vi "Check Status.vi"(0 "session in":T4[](array[typedef]) {"rx baseband session"."3630 session"."Address Space" items=["VXI/VME A16"=1, "VXI/VME A24"=2, "VXI/VME A32"=3, "VXI/VME A64"=4, "PXI Memory Allocations"=9, "PXI Configuration"=10, "PXI BAR0"=11, "PXI BAR1"=12, "PXI BAR2"=13, "PXI BAR3"=14, "PXI BAR4"=15, "PXI BAR5"=16]; "tx baseband session"."3610 session"."Address Space" items=["VXI/VME A16"=1, "VXI/VME A24"=2, "VXI/VME A32"=3, "VXI/VME A64"=4, "PXI Memory Allocations"=9, "PXI Configuration"=10, "PXI BAR0"=11, "PXI BAR1"=12, "PXI BAR2"=13, "PXI BAR3"=14, "PXI BAR4"=15, "PXI BAR5"=16]}, 11 "error in":errorcluster) -> (4 "session out":T4[](array[typedef]) {"rx baseband session"."3630 session"."Address Space" items=["VXI/VME A16"=1, "VXI/VME A24"=2, "VXI/VME A32"=3, "VXI/VME A64"=4, "PXI Memory Allocations"=9, "PXI Configuration"=10, "PXI BAR0"=11, "PXI BAR1"=12, "PXI BAR2"=13, "PXI BAR3"=14, "PXI BAR4"=15, "PXI BAR5"=16]; "tx baseband session"."3610 session"."Address Space" items=["VXI/VME A16"=1, "VXI/VME A24"=2, "VXI/VME A32"=3, "VXI/VME A64"=4, "PXI Memory Allocations"=9, "PXI Configuration"=10, "PXI BAR0"=11, "PXI BAR1"=12, "PXI BAR2"=13, "PXI BAR3"=14, "PXI BAR4"=15, "PXI BAR5"=16]}, 6 "rx status":T3(array[cluster]), 8 "tx status":T1(array[cluster]), 10 "dac alarms":T2[][](array[typedef]), 15 "error out":errorcluster)   [LabVIEW 2019, in "mmWave HW Control.lvlib"]
uses:
  Low-level/TypeDefs/Session.ctl
  <instrlib>/niMmWave/ni3620/Config/v1/Host/Public/High-Level/niMmWave Session.ctl
  <instrlib>/_niInstr/Register Bus/v0/Host/Public/Register Bus Session.ctl
  <instrlib>/_niInstr/Register Bus/v0/Host/Private/Session Data.ctl
  <instrlib>/niMmWave/ni3620/Config/v1/Host/Public/Typedefs/Board Information.ctl
  <instrlib>/niMmWave/ni3620/Config/v1/Host/Public/Typedefs/Hardware Revision.ctl
  <instrlib>/niMmWave/ni3620/Config/v1/Host/Public/Typedefs/Gain Mapping.ctl
  <instrlib>/niMmWave/ni3620/Config/v1/Host/Public/Typedefs/Correction Data.ctl
  <instrlib>/niMmWave/ni3620/Config/v1/Host/Public/Typedefs/Opera Characterization.ctl
  <instrlib>/niMmWave/ni3620/Config/v1/Host/Public/Corrections/Typedefs/Opera Characterization Main Header.ctl
  <instrlib>/niMmWave/ni3620/Config/v1/Host/Public/Corrections/Typedefs/Opera IF Board Information.ctl
  <instrlib>/niMmWave/ni3620/Config/v1/Host/Public/Corrections/Typedefs/Opera Characterization Instance Header.ctl
  <instrlib>/niMmWave/ni3620/Config/v1/Host/Public/Corrections/Typedefs/Opera Characterization Device Data Header.ctl
  <instrlib>/niMmWave/ni3620/Config/v1/Host/Public/Corrections/Typedefs/Opera LO Characterization Data Header.ctl
  <instrlib>/niMmWave/ni3620/Config/v1/Host/Public/Corrections/Typedefs/Opera IF Board Characterization Data Header.ctl
  <instrlib>/niMmWave/ni3620/Config/v1/Host/Public/Corrections/Typedefs/Opera Characterization Device Data.ctl
  <instrlib>/niMmWave/ni3620/Config/v1/Host/Public/Corrections/Typedefs/Opera LO2 Board Characterization Data.ctl
  <instrlib>/niMmWave/ni3620/Config/v1/Host/Public/Corrections/Typedefs/Opera LO Characterization Data.ctl
  <instrlib>/niMmWave/ni3620/Config/v1/Host/Public/Corrections/Typedefs/Opera IF Board Characterization Data.ctl
  <instrlib>/niMmWave/ni3620/Config/v1/Host/Public/Corrections/Typedefs/Opera IQ Impairment Data.ctl
  <instrlib>/niMmWave/ni3620/Config/v1/Host/Public/Typedefs/mmWave Adapter Session Data.ctl
  <instrlib>/niMmWave/ni3620/Config/v1/Host/Public/Typedefs/mmWave Adapter Data.ctl
  <instrlib>/niMmWave/ni3620/Config/v1/Host/Public/Typedefs/mmWave Adapter 2.ctl
  <instrlib>/niMmWave/ni3620/Config/v1/Shared/Typedefs/Subsystem ID.ctl
  <instrlib>/niMmWave/ni3620/Config/v1/Host/Public/Typedefs/mmWave Adapter Channel Information.ctl
  <instrlib>/niMmWave/ni3620/Config/v1/Host/Public/Typedefs/Temperature Coefficients.ctl
  <instrlib>/niMmWave/ni3620/Config/v1/Host/Public/Typedefs/mmWave Characterization.ctl
  <instrlib>/niMmWave/ni3620/Config/v1/Host/Public/Corrections/Typedefs/mmWave Characterization Main Header.ctl
  <instrlib>/niMmWave/ni3620/Config/v1/Host/Public/Corrections/Typedefs/mmWave Characterization Instance Header.ctl
  <instrlib>/niMmWave/ni3620/Config/v1/Host/Public/Typedefs/Session Cache.ctl
  <instrlib>/niMmWave/ni3620/Config/v1/Host/Public/Typedefs/LO2 settings cache.ctl
  <instrlib>/niMmWave/ni3620/Config/v1/Host/Public/Typedefs/LO2 source.ctl
  <instrlib>/niMmWave/ni3620/Config/v1/Host/Public/Typedefs/Desired and Coerced.ctl
  <instrlib>/niMmWave/ni3620/Config/v1/Host/Public/Typedefs/Export cache.ctl
  <instrlib>/niMmWave/ni3620/Config/v1/Host/Public/Typedefs/Path cache.ctl
  <instrlib>/niMmWave/ni3620/Config/v1/Host/Public/Typedefs/Daughterboard Type.ctl
  <instrlib>/niMmWave/ni3620/Config/v1/Host/Public/Typedefs/LO1 settings cache.ctl
  <instrlib>/niMmWave/ni3620/Config/v1/Host/Public/Typedefs/LO1 Source.ctl
  <instrlib>/niMmWave/ni3620/Config/v1/Host/Public/Typedefs/mmWave export cache.ctl
  <instrlib>/niMmWave/ni3620/Config/v1/Host/Private/Board/LO2/LO2 Board Configuration Cache.ctl
  <instrlib>/niMmWave/ni3620/Config/v1/Host/Public/Typedefs/reference clock routing settings.ctl
  <instrlib>/niMmWave/ni3620/Config/v1/Host/Public/Typedefs/LO2 routing settings.ctl
  <instrlib>/niMmWave/ni3620/Config/v1/Host/Private/Board/LO1/LO1 Board Configuration Cache.ctl
  <instrlib>/niMmWave/ni3620/Config/v1/Host/Public/Typedefs/LO1 source settings.ctl
  <instrlib>/niMmWave/ni3620/Config/v1/Host/Public/Typedefs/LO1 export settings.ctl
  <instrlib>/niMmWave/ni3620/Config/v1/Host/Public/Typedefs/LO1 mmWave settings.ctl
  Low-level/TypeDefs/Tx Baseband Session.ctl
  <instrlib>/niMmWave/ni3610 and ni3630/controls/public/Main Settings.ctl
  <vilib>/Instr/_visa.llb/VISA Register Access Address Space.ctl
  <instrlib>/niMmWave/ni3610 and ni3630/controls/public/Register Adresses.ctl
  <instrlib>/niMmWave/ni3610 and ni3630/controls/public/Base Card Type.ctl
  <instrlib>/niMmWave/ni3610 and ni3630/controls/private/IQ Card Revision.ctl
  <instrlib>/niMmWave/ni3610 and ni3630/controls/public/Board Capability.ctl
  Low-level/TypeDefs/Blank FPGA Reference.ctl
  Low-level/TypeDefs/Rx Baseband Session.ctl
  Low-level/TypeDefs/Hardware Configuration.ctl
  Low-level/TypeDefs/Direction.ctl
  Low-level/TypeDefs/Gain Ranging.ctl
  Low-level/TypeDefs/PXI Trigger Bus Info.ctl
  <instrlib>/niMmWave/ni3610 and ni3630/controls/public/DAC Alarms.ctl
  Low-level/TypeDefs/RX FPGA Reference.ctl
  <instrlib>/niMmWave/ni3610 and ni3630/controls/public/Converter Path Selector.ctl
  Low-level/TypeDefs/TX FPGA Reference.ctl
  <vilib>/rvi/errors/niLvFpgaAdjustHostInterfaceError.vi
  <vilib>/rvi/interface/nirviReadWriteControl/nirviReadWriteControl.xnode
  mmWave HW Control.lvlib
  NiFpgaLv.dll
  <vilib>/rvi/interface/Simulation/niFpgaSimulationCallBeginRW.vi
  <instrlib>/niMmWave/ni3610 and ni3630/ni3610_and_ni3630_Driver_Lib.lvlib
  <instrlib>/niMmWave/ni3620/Config/v1/Host/niMmWave Config v1 Host.lvlib
  <instrlib>/_niInstr/Register Bus/v0/Host/niInstr Register Bus v0 Host.lvlib
  <instrlib>/niMmWave/ni3620/Config/v1/Shared/niMmWave Config v1 Shared.lvlib
panel:
  # "Lane Number"
  # "0     1     2    3     4    5     6    7"
  # "Multiframe Alignment Error"
  # "Frame Alignment Error"
  # "Link Configuration Error"
  # "Elastic Buffer Overflow"
  # "Elastic Buffer Match Error"
  # "Code Group Synch. Error"
  # "8b/10b Not-in-Table Error"
  # "8b/10b Disparity Error"
  # "Lane Number"
  # "0     1     2    3     4    5     6    7"
  # "FIFO Write Error"
  # "FIFO Write Full"
  # "FIFO Read Error"
  # "FIFO Read Empty"
  # "Short Test Error"
  # "LOS Detect Alarm"
  # "SYSREF Alarms\n0      1      2     3"
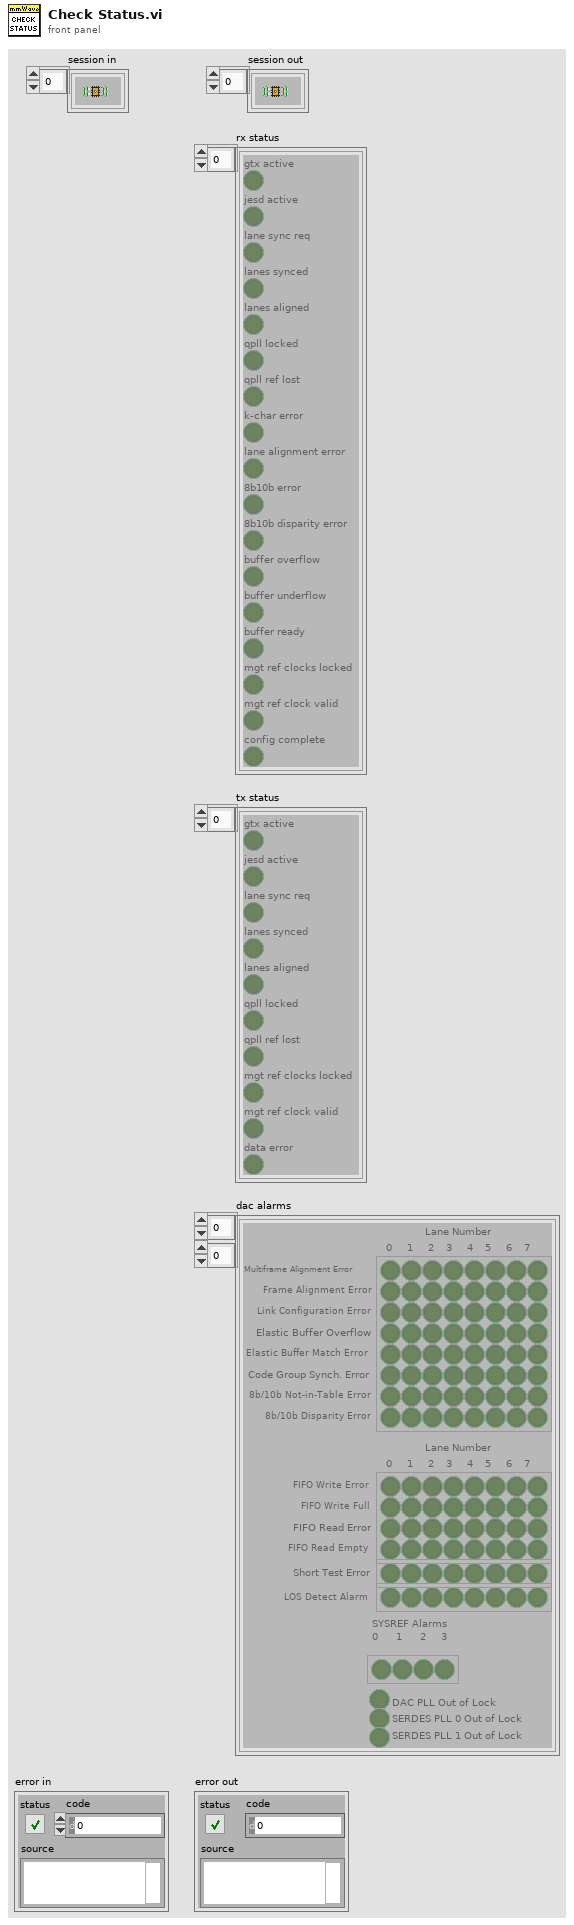
[diagram p1: front panel]
types:
  T1 = cluster{"gtx active":bool, "jesd active":bool, "lane sync req":bool, "lanes synced":bool, "lanes aligned":bool, "qpll locked":bool, "qpll ref lost":bool, "mgt ref clocks locked":bool, "mgt ref clock valid":bool, "data error":bool}[]
  T2 = typedef "ni3610_and_ni3630_Driver_Lib.lvlib/DAC Alarms.ctl" = cluster{"Lane Errors":bool[][], "FIFO Errors":bool[][], "Short Test Alarms":bool[], "LOS Alarms":bool[], "SYSREF Errors":bool[], "DAC38J84 PLL Out of Lock 3":bool, "DAC38J84 RW0 Out of Lock 3":bool, "DAC38J84 RW1 Out of Lock 3":bool}
  T3 = cluster{"gtx active":bool, "jesd active":bool, "lane sync req":bool, "lanes synced":bool, "lanes aligned":bool, "qpll locked":bool, "qpll ref lost":bool, "k-char error":bool, "lane alignment error":bool, "8b10b error":bool, "8b10b disparity error":bool, "buffer overflow":bool, "buffer underflow":bool, "buffer ready":bool, "mgt ref clocks locked":bool, "mgt ref clock valid":bool, "config complete":bool}[]
  T4 = typedef "Session.ctl" = cluster{"3620 session":refnum<queue>, "tx baseband session":T5, "rx baseband session":T13, "tx gain (dB)":dbl, "rx gain (dB)":dbl, "hardware configuration":T14, "gain ranging":T16[], "pxi trigger bus information":T17}
  T5 = typedef "Tx Baseband Session.ctl" = cluster{"3610 session":T6, "7902 reference":T12}
  T6 = typedef "ni3610_and_ni3630_Driver_Lib.lvlib/Main Settings.ctl" = cluster{"VISA resource name":refnum<visa-resource-name>, "Address Space":T7, "window_offset":u32, "register_addresses":T8, "required_MM_fpga_version":cluster{"signature":u32, "hardware":u32, "current revision":u32, "oldest revision":u32}, "CPLD Oldest Compat Version ":cluster{"hardware":u32, "CPLD firmware":u32}, "MM_FPGA_image_location":string, "is_init":bool, "card_type":T9, "DacLmkConfigFileName":string, "AdcLmkConfigFileName":string, "AdcConfigFileName":string, "DacConfigFileName_RevA":string, "DacConfigFileName_RevB":string, "Mulde hardware revision":u8, "bypass DAC PLL\n":bool, "IQ Card Revision":T10, "board capability":T11}
  T7 = typedef "VISA Register Access Address Space.ctl" = u16
  T8 = typedef "ni3610_and_ni3630_Driver_Lib.lvlib/Register Adresses.ctl" = cluster{"MM based Registers":cluster{"Revision":u32, "OldestCompatRev":u32, "signature":u32, "scratch":u32, "LedControl":u32, "BoardHwRev":u32, "BoardControl":u32, "ThermalStatus":u32, "BasebandStatus":u32, "BasebandControl":u32, "BasebandAuxSetup":u32, "BasebandAuxStatus":u32, "LmkSyncOutSetup":u32, " AdcSyncOutSetup":u32, " InjSyncOutSetup":u32, " PxiTrig0OutSetup":u32, " PxiTrig1OutSetup":u32, " PxiTrig2OutSetup":u32, " PxiTrig3OutSetup":u32, " PxiTrig4OutSetup":u32, " PxiTrig5OutSetup":u32, " PxiTrig6OutSetup":u32, " PxiTrig7OutSetup":u32}, "CPLD based Registers":cluster{"SlaveSignature":u32, "SlaveRevision":u32, "SlaveOldestCompatRev":u32, "SlaveScratch":u32, "SlaveSetup":u32, "SlaveStatus":u32, "IDacReg_offset":u32, "LMKRegGrp0_offset":u32, "QDacReg_offset":u32, "BrdTempSensorVal":u32, "TempSensorPowerDown":u32, "GPIOReg_offset":u32, "IAdcReg_offset":u32, "QAdcReg_offset":u32, "LMKRegGrp1_offset":u32, "QadcTempSensorVal":u32, "IadcTempSensorVal":u32, "RevisionReg":u32, "VcxoReg":u32, "CpldStatusReg":u32, "PowerReg":u32, "VBiasEnReg":u32, "ExtRefOeReg":u32, "QdacCtrlReg":u32, "QdacStatusReg":u32, "IdacCtrlReg":u32, "IdacStatusReg":u32, "QdacJtagIn":u32, "QdacJtagOut":u32, "IdacJtagIn":u32, "IdacJtagOut":u32, "IqDcSetupReg":u32, "QadcStatusReg":u32, "IadcStatusReg":u32, "BrdSetupReg":u32, "IqDcRevisionReg":u32, "PllStatusReg":u32, "EndpointScratchReg":u32, "AdcSyncCfgReg":u32, "IqCardOpampReg":u32}, "CPLD Register Offset":u32, "MM  Register Offset":u32, " PxiTrig0OutSetup":u32}
  T9 = typedef "ni3610_and_ni3630_Driver_Lib.lvlib/Base Card Type.ctl" = enum16{"unspecified", "ADC", "DAC"}
  T10 = typedef "ni3610_and_ni3630_Driver_Lib.lvlib/IQ Card Revision.ctl" = enum16{"RevA", "RevB", "RevC", "RevD"}
  T11 = typedef "ni3610_and_ni3630_Driver_Lib.lvlib/Board Capability.ctl" = cluster{"baseband sync":enum16{"no baseband sync", "baseband sync"}}
  T12 = typedef "Blank FPGA Reference.ctl" = refnum<k20>
  T13 = typedef "Rx Baseband Session.ctl" = cluster{"3630 session":T6, "7902 reference":T12}
  T14 = typedef "Hardware Configuration.ctl" = cluster{"direction":T15, "baseband only":bool}
  T15 = typedef "Direction.ctl" = enum16{"Transceiver", "Receiver", "Transmitter"}
  T16 = typedef "Gain Ranging.ctl" = cluster{"gain ranging active scope":string, "gain ranging stream session":refnum<k20>}
  T17 = typedef "PXI Trigger Bus Info.ctl" = cluster{"chassis resource name":refnum<visa-resource-name>, "7902R (TX)":i16, "3610 (TX)":i16, "3620 (IF)":i16, "3630 (RX)":i16, "7902R (RX)":i16}
  T18 = cluster{"gtx active":bool, "jesd active":bool, "lane sync req":bool, "lanes synced":bool, "lanes aligned":bool, "qpll locked":bool, "qpll ref lost":bool, "k-char error":bool, "lane alignment error":bool, "8b10b error":bool, "8b10b disparity error":bool, "buffer overflow":bool, "buffer underflow":bool, "buffer ready":bool, "mgt ref clocks locked":bool, "mgt ref clock valid":bool, "config complete":bool}
  T19 = typedef "RX FPGA Reference.ctl" = refnum<k20>
  T20 = cluster{"gtx active":bool, "jesd active":bool, "lane sync req":bool, "lanes synced":bool, "lanes aligned":bool, "qpll locked":bool, "qpll ref lost":bool, "mgt ref clocks locked":bool, "mgt ref clock valid":bool, "data error":bool}
  T21 = typedef "TX FPGA Reference.ctl" = refnum<k20>
  T22 = typedef "ni3610_and_ni3630_Driver_Lib.lvlib/Converter Path Selector.ctl" = enum16{"I-path device", "Q-path device"}
  T23 = typedef "ni3610_and_ni3630_Driver_Lib.lvlib/ADC Status.ctl" = cluster{"JESD Link Up":bool, "JESD Sync Status":bool, "JESD Realigned":bool, "JESD Aligned":bool, "Powered Down":bool, "Gain_FS[mVp-p]":dbl, "Offset_FS[mV]":dbl}
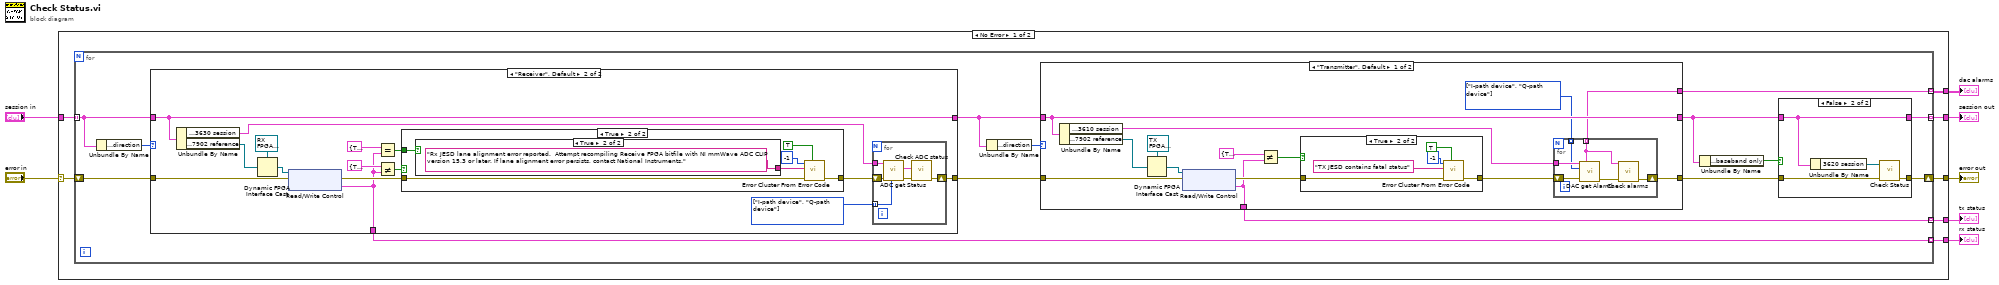
[diagram p0: block diagram]
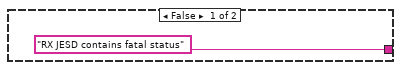
[diagram p4: hidden frame]
diagram:
  n1 = case shown="No Error" "error in" {
    selector: "error in" -> [w12 w95]
    tunnel: "session in" -> [w14 w96]
    tunnel: [w13 w96] -> w6
    tunnel: [w11 w95] -> w4
    tunnel: [w10 _] -> w3
    tunnel: [w9 _] -> w1
    tunnel: [w8 _] -> w2
    frame No Error {
      n2 = for {
        tunnel: w14 -> [w26] mode=indexing
        tunnel: [w15] -> w13 mode=indexing
        shift-right: [w19] -> w11
        shift-left: w12 -> [w28]
        tunnel: [w27] -> w10 mode=indexing
        tunnel: [w21] -> w9 mode=indexing
        tunnel: [w20] -> w8 mode=indexing
        n3 = Unbundle By Name(w26) -> ("hardware configuration.direction"=w25:T15)
        n4 = case shown="\"Receiver\", Default" w25 {
          tunnel: w26 -> [w30 w41]
          tunnel: w28 -> [w29 w45]
          tunnel: [w29 w37] -> w24
          tunnel: [_ w32] -> w27
          tunnel: [w30 w41] -> w22
          frame "Transmitter" {
          }
          frame "Receiver", Default {
            w35 = T22[] [enum."I-path device", enum."Q-path device"] items=["I-path device", "Q-path device"]
            n5 = Unbundle By Name(w41) -> ("rx baseband session.3630 session"=w36:T6, "rx baseband session.7902 reference"=w44:T12)
            n6 = Dynamic FPGA Interface Cast(Session In=T19 refnum ("fpga reference"), Type=w44) -> (Session Out=w42:T19)
            n7 = xnode "Read/Write Control"("FPGA VI Reference In"=w42, "error in"=w45) -> ("error out"=w40:errorcluster, "rxjesd.status"=w32:T18)  [unwired: 1 out]
            n8 = Equal?(x=T18 {"gtx active"=TRUE, "jesd active"=TRUE, "lane sync req"=FALSE, "lanes synced"=TRUE, "lanes aligned"=TRUE, "qpll locked"=TRUE, "qpll ref lost"=FALSE, "k-char error"=FALSE, "lane alignment error"=TRUE, "8b10b error"=FALSE, "8b10b disparity error"=FALSE, "buffer overflow"=FALSE, "buffer underflow"=FALSE, "buffer ready"=TRUE, "mgt ref clocks locked"=TRUE, "mgt ref clock valid"=TRUE, "config complete"=TRUE} ("rxjesd.status"), y=w32) -> (x = y?=w31:bool)
            n9 = Not Equal?(x=T18 {"gtx active"=TRUE, "jesd active"=TRUE, "lane sync req"=FALSE, "lanes synced"=TRUE, "lanes aligned"=TRUE, "qpll locked"=TRUE, "qpll ref lost"=FALSE, "k-char error"=FALSE, "lane alignment error"=FALSE, "8b10b error"=FALSE, "8b10b disparity error"=FALSE, "buffer overflow"=FALSE, "buffer underflow"=FALSE, "buffer ready"=TRUE, "mgt ref clocks locked"=TRUE, "mgt ref clock valid"=TRUE, "config complete"=TRUE} ("rxjesd.status"), y=w32) -> (x != y?=w39:bool)
            n10 = case shown="True" w39 {
              tunnel: w40 -> [w46 w52]
              tunnel: [w46 w51] -> w38
              tunnel: w31 -> [_ w47]
              frame False {
              }
              frame True {
                n11 = case shown="True" w47 {
                  tunnel: ["RX JESD contains fatal status" ("error message (\"\")") "Rx JESD lane alignment error reported.  Attempt recompiling Receive FPGA bitfile with NI mmWave ADC CLIP version 15.3 or later. If lane alignment error persists, contact National Instruments." ("error message (\"\")")] -> w48
                  frame False {
                  }
                  frame True {
                  }
                }
                n12 = call <vilib>:"Error Cluster From Error Code.vi"("show call chain? (False)"=TRUE, "error in (no error)"=w52, "error message (\"\")"=w48, "error code (0)"=-1 ("specific error code to clear (0: all)")) -> ("error out"=w51:errorcluster)  [unwired: 5 in]
              }
            }
            n13 = for {
              tunnel: w36 -> [w56]
              shift-right: [w58] -> w37
              shift-left: w38 -> [w60]
              tunnel: w35 -> [w55] mode=indexing
              n14 = call <instrlib>:"ADC get Status.vi"("Converter Selection"=w55, "error in"=w60, "Board Settings in"=w56) -> ("error out"=w59:errorcluster, "ADC Status"=w57:T23)  [unwired: 6 in, 1 out]
              n15 = call "Check ADC status.vi"("ADC Status"=w57, "error in (no error)"=w59) -> ("error out"=w58:errorcluster)  [unwired: 13 in]
            }
          }
        }
        n16 = Unbundle By Name(w22) -> ("hardware configuration.direction"=w23:T15)
        n17 = case shown="\"Transmitter\", Default" w23 {
          tunnel: w24 -> [w77 w93]
          tunnel: w22 -> [w76 w94]
          tunnel: [w71 _] -> w21
          tunnel: [w76 w94] -> w16
          tunnel: [w75 w93] -> w18
          tunnel: [w73 _] -> w20
          frame "Transmitter", Default {
            w74 = T22[] [enum."I-path device", enum."Q-path device"] items=["I-path device", "Q-path device"]
            n18 = Unbundle By Name(w76) -> ("tx baseband session.3610 session"=w68:T6, "tx baseband session.7902 reference"=w79:T12)
            n19 = Dynamic FPGA Interface Cast(Session In=T21 refnum ("Refnum in"), Type=w79) -> (Session Out=w78:T21)
            n20 = xnode "Read/Write Control"("FPGA VI Reference In"=w78, "error in"=w77) -> ("error out"=w72:errorcluster, "txjesd.status"=w71:T20)  [unwired: 1 out]
            n21 = Not Equal?(x=T20 {"gtx active"=TRUE, "jesd active"=TRUE, "lane sync req"=FALSE, "lanes synced"=TRUE, "lanes aligned"=TRUE, "qpll locked"=TRUE, "qpll ref lost"=FALSE, "mgt ref clocks locked"=TRUE, "mgt ref clock valid"=TRUE, "data error"=FALSE}, y=w71) -> (x != y?=w69:bool)
            n22 = case shown="True" w69 {
              tunnel: w72 -> [w81 w86]
              tunnel: [w81 w85] -> w67
              frame False {
              }
              frame True {
                n23 = call <vilib>:"Error Cluster From Error Code.vi"("show call chain? (False)"=TRUE, "error in (no error)"=w86, "error message (\"\")"="TX JESD contains fatal status" ("error message (\"\")"), "error code (0)"=-1 ("specific error code to clear (0: all)")) -> ("error out"=w85:errorcluster)  [unwired: 5 in]
              }
            }
            n24 = for {
              shift-right: [w88] -> w75
              shift-left: w67 -> [w92]
              tunnel: w68 -> [w91]
              tunnel: w74 -> [w90] mode=indexing
              tunnel: [w87] -> w73 mode=indexing
              n25 = call <instrlib>:"DAC get Alarms.vi"("Board Settings in"=w91, "Converter Path Selection"=w90, "error in"=w92) -> ("alarms"=w87:T2, "error out"=w89:errorcluster)  [unwired: 14 in, 9 out]
              n26 = call "Check alarms.vi"("alarms"=w87, "error in (no error)"=w89) -> ("error out"=w88:errorcluster)  [unwired: 13 in]
            }
          }
          frame "Receiver" {
          }
        }
        n27 = Unbundle By Name(w16) -> ("hardware configuration.baseband only"=w17:bool)
        n28 = case shown="False" w17 {
          tunnel: [w62 w66] -> w19
          tunnel: w18 -> [w62 w65]
          tunnel: w16 -> [w61 w63]
          tunnel: [w61 w63] -> w15
          frame True {
          }
          frame False {
            n29 = Unbundle By Name(w63) -> ("3620 session"=w64:refnum<queue>)
            n30 = call <instrlib>:"Check Status.vi"("session in"=w64, "error in"=w65) -> ("error out"=w66:errorcluster)  [unwired: 12 in, 1 out]
          }
        }
      }
    }
    frame Error {
    }
  }
  "session out" <- w6
  "error out" <- w4
  "rx status" <- w3
  "dac alarms" <- w2
  "tx status" <- w1
